vi "Sub VI Temperature.vi"() -> ()   [LabVIEW 2023]
panel:
  out "Fahrenheit":dbl(slide) scale=0.0..2000.0
  in  "Celsius":dbl(slide) scale=0.0..1000.0
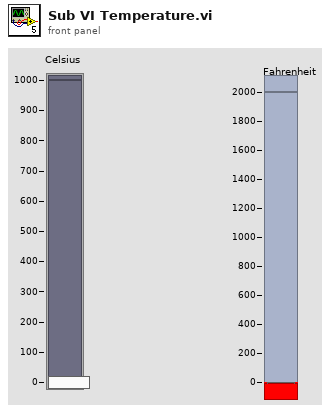
[diagram p1: front panel]
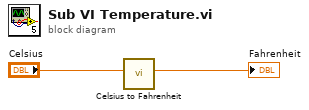
[diagram p0: block diagram]
diagram:
  n1 = call "Celsius to Fahrenheit.vi"("Celsius"="Celsius") -> ("Fahrenheit"=→"Fahrenheit":dbl)  [unwired: 10 in]
